vi "10-type_analog.vi"(2 "this":i32, 3 "button":i32, 4 "Cluster":T1={"Auto1"=TRUE, "Auto2"=TRUE, "Rel1"=TRUE, "Rel2"=TRUE, "Filt1"=TRUE, "Filt2"=TRUE, "Rate"=enum."Slow", "Range1"=enum."10mV", "Range2"=enum."100mV", "Filt3"=TRUE, "Filt4"=TRUE, "Rel temp 1"=TRUE, "Analog1"=FALSE, "Analog2"=FALSE, "Analog temp 1"=FALSE, "Digital1"=TRUE, "Digital2"=TRUE, "Digital temp 1 "=TRUE, "Window1"=enum."0,01%", "Window2"=enum."0,01%", "Window temp 1"=enum."0,01%", "RDGS1"="010", "RDGS2"="010", "RDGS temp 1"="010", "Type_type1"=TRUE, "Type_type2"=TRUE, "Type_type temp 1"=TRUE, "LSync"=FALSE, "Unit"=enum."C", "Sens"=TRUE, "Type tcoupl"=enum."J", "Junc"=TRUE, "prevState"=0, "Rel temp 2"=TRUE, "Analog temp 2"=FALSE, "Digital temp 2"=TRUE, "Type_type temp 2"=TRUE, "RDGS temp 2"="010", "Window temp 2"=enum."0,01%", "address"="0"}) -> (0 "next state":i32, 1 "Cluster 2":T1)   [LabVIEW 2017]
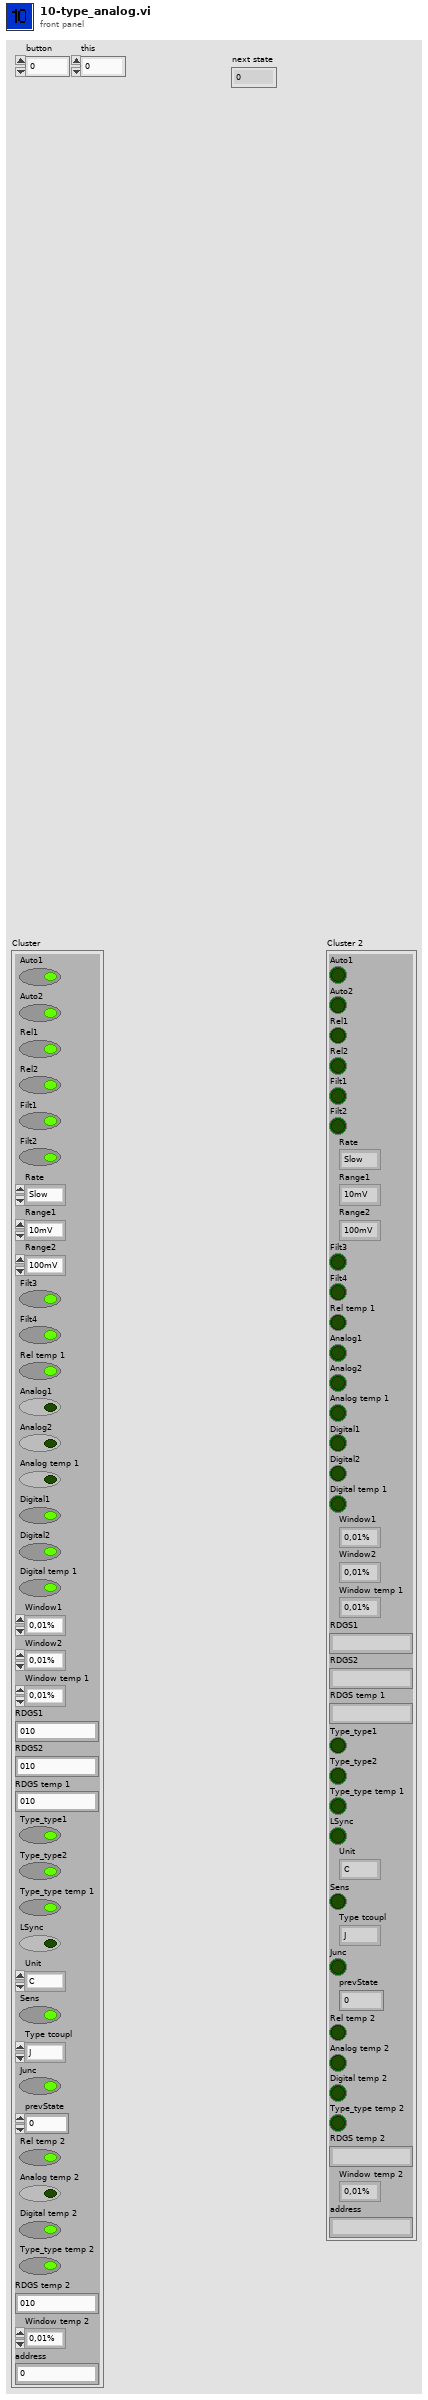
[diagram p1: front panel]
types:
  T1 = cluster{"Auto1":bool, "Auto2":bool, "Rel1":bool, "Rel2":bool, "Filt1":bool, "Filt2":bool, "Rate":enum16{"Slow", "Med", "Fast"}, "Range1":enum16{"10mV", "100mV", "1V", "10V", "100V"}, "Range2":enum16{"100mV", "1V", "10V"}, "Filt3":bool, "Filt4":bool, "Rel temp 1":bool, "Analog1":bool, "Analog2":bool, "Analog temp 1":bool, "Digital1":bool, "Digital2":bool, "Digital temp 1 ":bool, "Window1":enum16{"0,01%", "0,1%", "1%", "10%", "None"}, "Window2":enum16{"0,01%", "0,1%", "1%", "10%", "None"}, "Window temp 1":enum16{"0,01%", "0,1%", "1%", "10%", "None"}, "RDGS1":string, "RDGS2":string, "RDGS temp 1":string, "Type_type1":bool, "Type_type2":bool, "Type_type temp 1":bool, "LSync":bool, "Unit":enum16{"C", "K", "F"}, "Sens":bool, "Type tcoupl":enum16{"J", "K", "T", "E", "R", "S", "B", "N"}, "Junc":bool, "prevState":i32, "Rel temp 2":bool, "Analog temp 2":bool, "Digital temp 2":bool, "Type_type temp 2":bool, "RDGS temp 2":string, "Window temp 2":enum16{"0,01%", "0,1%", "1%", "10%", "None"}, "address":string}
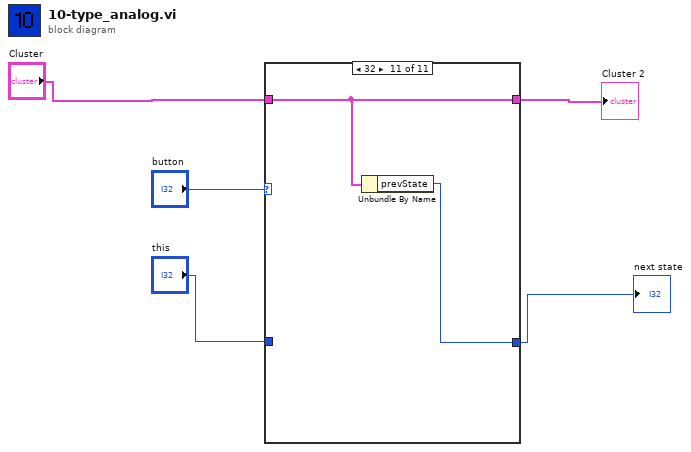
[diagram p0: block diagram]
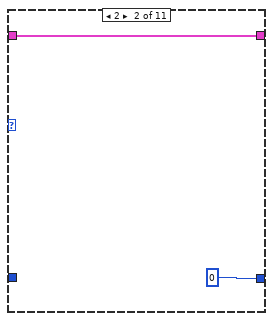
[diagram p3: hidden frame]
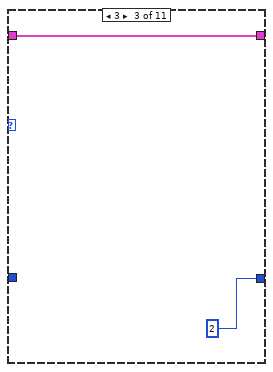
[diagram p4: hidden frame]
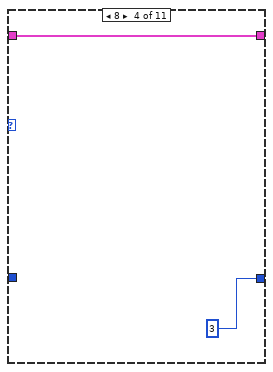
[diagram p5: hidden frame]
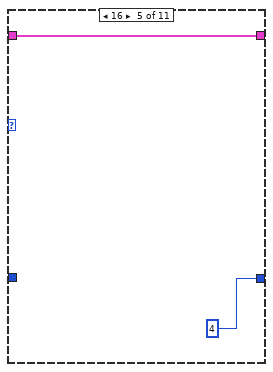
[diagram p6: hidden frame]
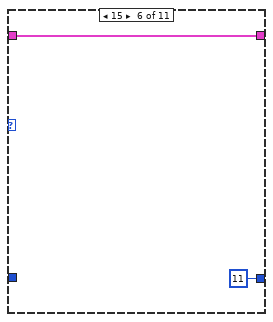
[diagram p7: hidden frame]
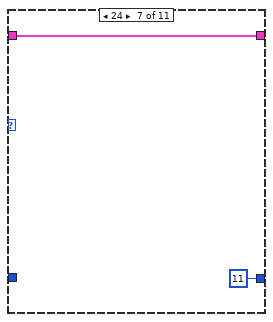
[diagram p8: hidden frame]
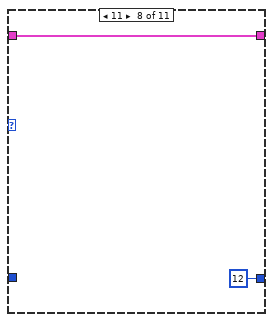
[diagram p9: hidden frame]
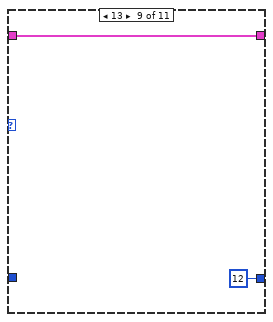
[diagram p10: hidden frame]
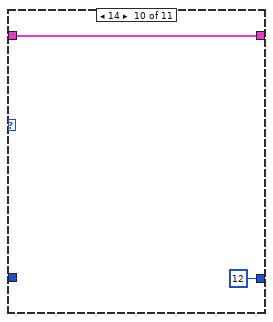
[diagram p11: hidden frame]
diagram:
  n1 = case shown="32" "button" {
    tunnel: [w6 0 ("this") 2 3 4 11 ("this") 11 ("this") 12 ("this") 12 ("this") 12 ("this") w26] -> w3
    tunnel: "this" -> [w6 _ _ _ _ _ _ _ _ _ _]
    tunnel: "Cluster" -> [w7 w9 w10 w12 w14 w17 w19 w21 w22 w25 w27]
    tunnel: [w7 w9 w10 w12 w14 w17 w19 w21 w22 w25 w27] -> w1
    frame Default {
    }
    frame 2 {
    }
    frame 3 {
    }
    frame 8 {
    }
    frame 16 {
    }
    frame 15 {
    }
    frame 24 {
    }
    frame 11 {
    }
    frame 13 {
    }
    frame 14 {
    }
    frame 32 {
      n2 = Unbundle By Name(w27) -> ("prevState"=w26:i32)
    }
  }
  "next state" <- w3
  "Cluster 2" <- w1
